vi "random number 2.vi"() -> ()   [LabVIEW 2012]
panel:
  out "output":dbl
  out "Array":dbl[](array[numeric])
  out "Counter":i32
  # "count"
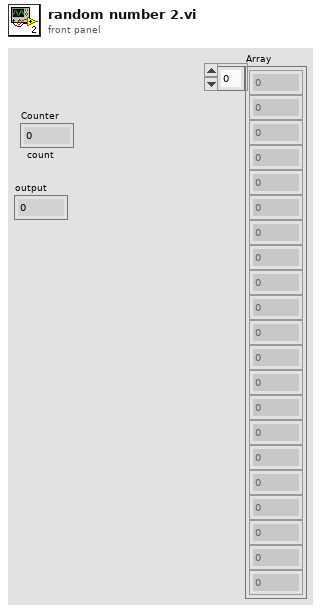
[diagram p1: front panel]
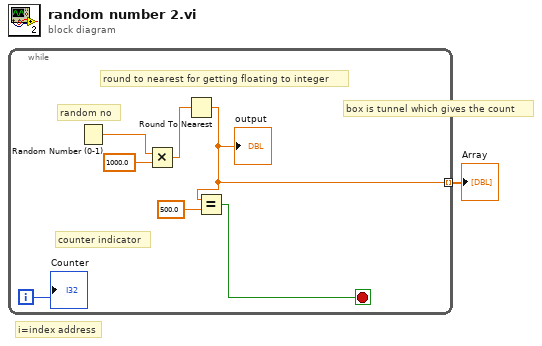
[diagram p0: block diagram]
diagram:
  # "box is tunnel which gives the count"
  # "i=index address"
  n1 = while {
    tunnel: [w2] -> w1 mode=indexing
    i -> [w4]
    stop <- w6 stop-if-true
    # "random no"
    # "counter indicator"
    # "round to nearest for getting floating to integer"
    n2 = Random Number (0-1)() -> (number: 0 to 1=w7:dbl)
    n3 = Multiply(x=w7, y=1000.0) -> (x*y=w3:dbl)
    n4 = Round To Nearest(number=w3) -> (nearest integer value=w2:dbl)
    "output" <- w2
    n5 = Equal?(x=w2, y=500.0) -> (x = y?=w6:bool)
    "Counter" <- w4
  }
  "Array" <- w1
